vi "Pipes.vi"(7 "Action":enum16{"Initialize", "Update"}(ring), 8 "error in (no error)":errorcluster, 10 "Variables":refnum<vi>[](array[refnum]), 11 "Pipes":refnum<vi>[](array[refnum])) -> (0 "error out":errorcluster)   [LabVIEW 2022 SP3, in "Pipes.lvlib"]
uses:
  Pipes.lvlib
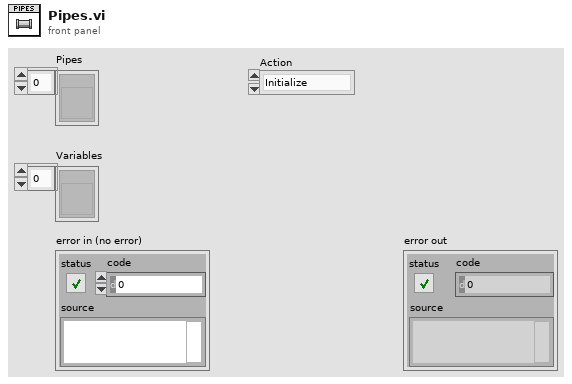
[diagram p1: front panel]
types:
  T1 = typedef "Pipes.lvlib/Pipe.ctl" = cluster{"Clone Idx":i32, "Defs":T2[]}
  T2 = typedef "Pipes.lvlib/Pipe Definition.ctl" = cluster{"Clone Idx":i32, "Color":u32, "Types":T3[], "Values":dbl[]}
  T3 = typedef "Pipes.lvlib/Token Type.ctl" = enum8{"INVALID", "NOT", "AND", "OR", "EE", "NE", "LT", "GT", "LTE", "GTE", "PLUS", "MINUS", "MULTIPLY", "DIVIDE", "MODULUS", "LPAREN", "RPAREN", "LITERAL", "IDENTIFIER", "DEFINITION"}
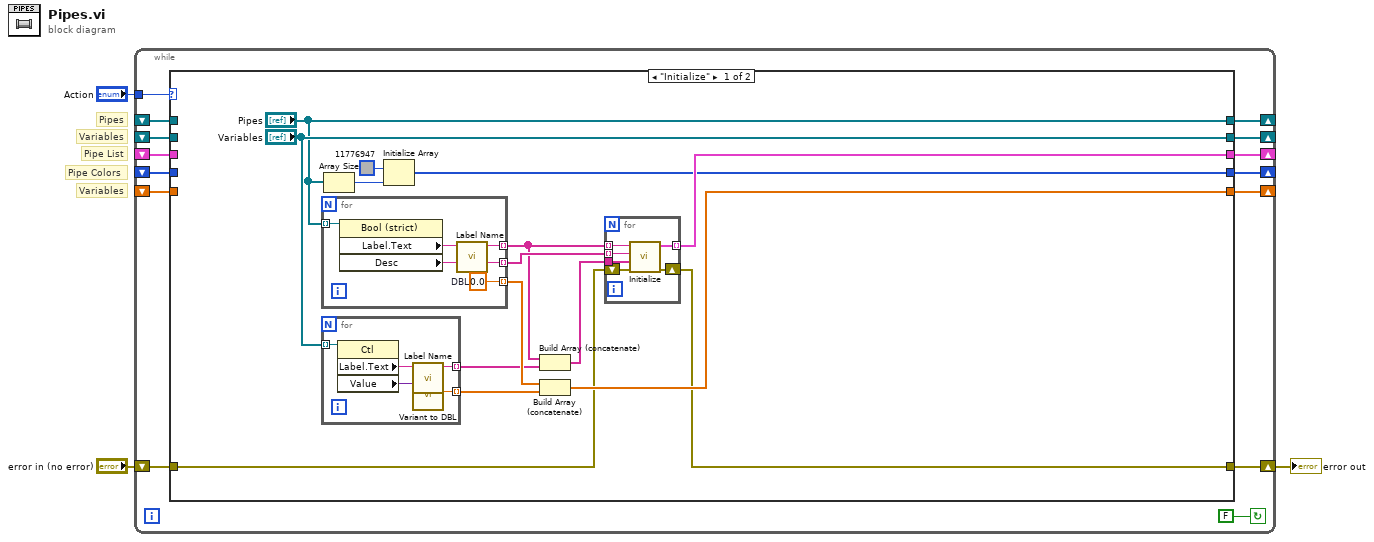
[diagram p0: block diagram]
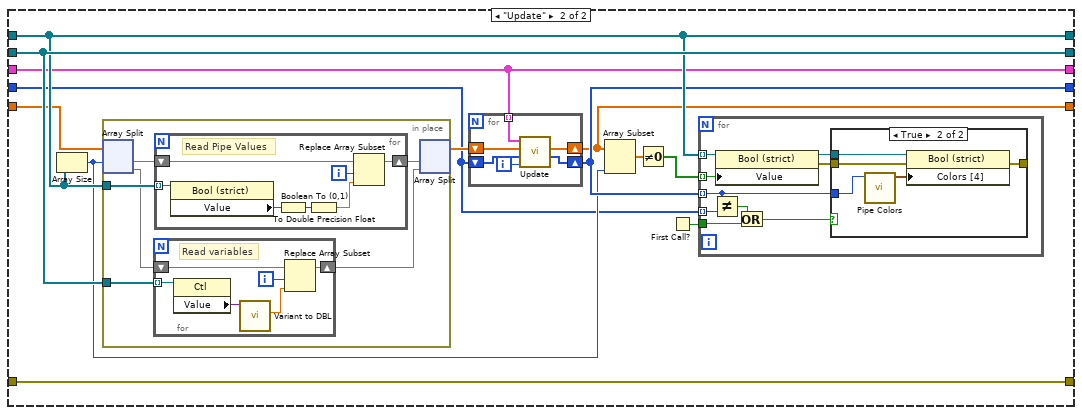
[diagram p2: hidden frame]
diagram:
  # "Variables"
  # "Pipe Colors"
  # "Pipe List"
  # "Variables"
  # "Pipes"
  n1 = while {
    shift-right: [w17] -> w3
    shift-left: "error in (no error)" -> [w16]
    tunnel: "Action" -> [w14]
    shift-right: [w13] -> _
    shift-left: _ -> [w10]
    shift-right: [w12] -> _
    shift-left: _ -> [w11]
    shift-right: [w8] -> _
    shift-left: _ -> [w9]
    shift-right: [w7] -> _
    shift-left: _ -> [w6]
    shift-right: [w5] -> _
    shift-left: _ -> [w4]
    stop <- FALSE continue-if-true
    n2 = case shown="\"Initialize\"" w14 {
      tunnel: [w19 w61] -> w17
      tunnel: w16 -> [w18 w61]
      tunnel: ["Pipes" w59] -> w13
      tunnel: ["Variables" w60] -> w12
      tunnel: w11 -> [_ w60]
      tunnel: w10 -> [_ w59]
      tunnel: w9 -> [_ w56]
      tunnel: [w30 w56] -> w8
      tunnel: [w28 w55] -> w7
      tunnel: w6 -> [_ w50]
      tunnel: [w20 w54] -> w5
      tunnel: w4 -> [_ w58]
      frame "Initialize" {
        n3 = for {
          tunnel: "Pipes" -> [w48] mode=indexing
          tunnel: [w44] -> w31 mode=indexing
          tunnel: [w47] -> w27 mode=indexing
          tunnel: [w45] -> w24 mode=indexing
          w47 = 0.0  # DBL
          n4 = property class="Bool (strict)"(reference=w48) -> ("Label.Text"=w46:string, "Desc"=w44:string)  [unwired: 1 in, 2 out]
          n5 = call "Label Name.vi"("Label Text"=w46) -> ("Variable Name"=w45:string)  [unwired: 10 in]
        }
        n6 = for {
          tunnel: "Variables" -> [w43] mode=indexing
          tunnel: [w41] -> w26 mode=indexing
          tunnel: [w39] -> w25 mode=indexing
          n7 = property class="Ctl"(reference=w43) -> ("Label.Text"=w42:string, "Value"=w40:variant)  [unwired: 1 in, 2 out]
          n8 = call "Label Name.vi"("Label Text"=w42) -> ("Variable Name"=w41:string)  [unwired: 10 in]
          n9 = call "Variant to DBL.vi"("Variant"=w40) -> ("Value as DBL"=w39:dbl)  [unwired: 9 in, 1 out]
        }
        n10 = Array Size(array="Pipes") -> (size(s)=w21:i32)
        n11 = Initialize Array(u32 11776947, w21) -> (w28:u32[])
        n12 = Build Array (concatenate)(w24, w26) -> (w23:string[])
        n13 = Build Array (concatenate)(w27, w25) -> (w20:dbl[])
        n14 = for {
          tunnel: w31 -> [w38] mode=indexing
          tunnel: [w37] -> w30 mode=indexing
          tunnel: w24 -> [w36] mode=indexing
          tunnel: w23 -> [w35]
          shift-right: [w33] -> w19
          shift-left: w18 -> [w34]
          n15 = call "Initialize.vi"("error in (no error)"=w34, "Variable Names"=w35, "Description"=w38, "Pipe Name"=w36) -> ("error out"=w33:errorcluster, "Pipe"=w37:T1)  [unwired: 6 in]
        }
      }
      frame "Update" {
        n16 = Array Size(array=w59) -> (size(s)=w53:i32)
        n17 = in-place {
          in-place-border: w60 -> [w73]
          in-place-border: w59 -> [w72]
          n18 = in-place-split #1(w58, w53) -> (w71:dbl[], w69:dbl[])
          n19 = for {
            tunnel: w73 -> [w86] mode=indexing
            shift-right: [w81] -> w68
            shift-left: w69 -> [w83]
            i -> [w82]
            # "Read variables"
            n20 = property class="Ctl"(reference=w86) -> ("Value"=w85:variant)  [unwired: 1 in, 2 out]
            n21 = call "Variant to DBL.vi"("Variant"=w85) -> ("Value as DBL"=w84:dbl)  [unwired: 9 in, 1 out]
            n22 = Replace Array Subset(array=w83, new element=w84, index=w82) -> (w81:dbl[])
          }
          n23 = for {
            tunnel: w72 -> [w80] mode=indexing
            shift-right: [w77] -> w70
            shift-left: w71 -> [w78]
            i -> [w76]
            # "Read Pipe Values"
            n24 = property class="Bool (strict)"(reference=w80) -> ("Value"=w79:bool)  [unwired: 1 in, 2 out]
            n25 = Boolean To (0,1)(Boolean=w79) -> (0, 1=w75:i16)
            n26 = To Double Precision Float(number=w75) -> (double precision float=w74:dbl)
            n27 = Replace Array Subset(array=w78, new element=w74, index=w76) -> (w77:dbl[])
          }
          n28 = in-place-split #1(w70, w68) -> (w57:dbl[])  [unwired: 1 out]
        }
        n29 = for {
          shift-right: [w64] -> w54
          shift-left: w57 -> [w65]
          shift-right: [w62] -> w55
          shift-left: w50 -> [w63]
          tunnel: w56 -> [w66] mode=indexing
          i -> [w67]
          n30 = call "Update.vi"("Index"=w67, "Pipe Colors in"=w63, "Values in"=w65, "Pipe in"=w66) -> ("Pipe Colors out"=w62:u32[], "Values out"=w64:dbl[])  [unwired: 6 in]
        }
        n31 = Array Subset(array=w54, length=w53) -> (w52:dbl[])  [unwired: 1 in]
        n32 = Not Equal To 0?(x=w52) -> (x != 0?=w51:bool[])
        n33 = First Call?() -> (First Call?: T/F=w49:bool)
        n34 = for {
          tunnel: w59 -> [w95] mode=indexing
          tunnel: w51 -> [w94] mode=indexing
          tunnel: w55 -> [w92] mode=indexing
          tunnel: w50 -> [w90] mode=indexing
          tunnel: w49 -> [w88]
          n35 = Not Equal?(x=w92, y=w90) -> (x != y?=w91:bool)
          n36 = property class="Bool (strict)"(reference=w95, "Value"=w94) -> (reference out=w93:refnum<vi>, error out=w87:errorcluster)  [unwired: 1 in]
          n37 = Or(x=w91, y=w88) -> (x .or. y?=w89:bool)
          n38 = case shown="True" w89 {
            tunnel: w92 -> [_ w101]
            tunnel: w93 -> [_ w100]
            tunnel: w87 -> [w96 w98]
            tunnel: [w96 w97] -> _
            frame False {
            }
            frame True {
              n39 = call "Pipe Colors.vi"("True Color"=w101) -> ("Colors[4]"=w99:cluster{"FG":u32, "BG":u32}[])  [unwired: 10 in]
              n40 = property class="Bool (strict)"(reference=w100, error in=w98, "Colors [4]"=w99) -> (error out=w97:errorcluster)  [unwired: 1 out]
            }
          }
        }
      }
    }
  }
  "error out" <- w3
